vi "CRYUpdate Curve Name of All Steps.vi"(0 "Start Index":i32, 1 "sOption":string, 5 "End Index":i32) -> ()   [LabVIEW 2013]
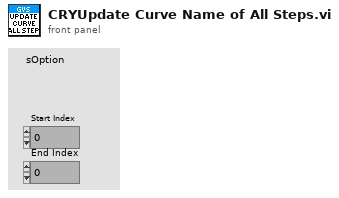
[diagram p1: front panel]
types:
  T1 = typedef "CRYStep.ctl" = cluster{"No.VI":i32, "Category":string, "StepName":string, "Seq setup flattened":string, "Comment":string, "Steps config.":bool[], "Jump config":i32[], "Start":dbl, "Increment":dbl, "Name":string, "Unit":string, "Y data":u16, "Y prefix":string, "Y dB ref":dbl, "Y unit":string, "Repeat State Array":cluster{"Start":dbl, "Increment":dbl, "Count":i32, "Num":i32}[]}
  T2 = enum16{"Curves", "Values", "Results", "WFM", "All"}
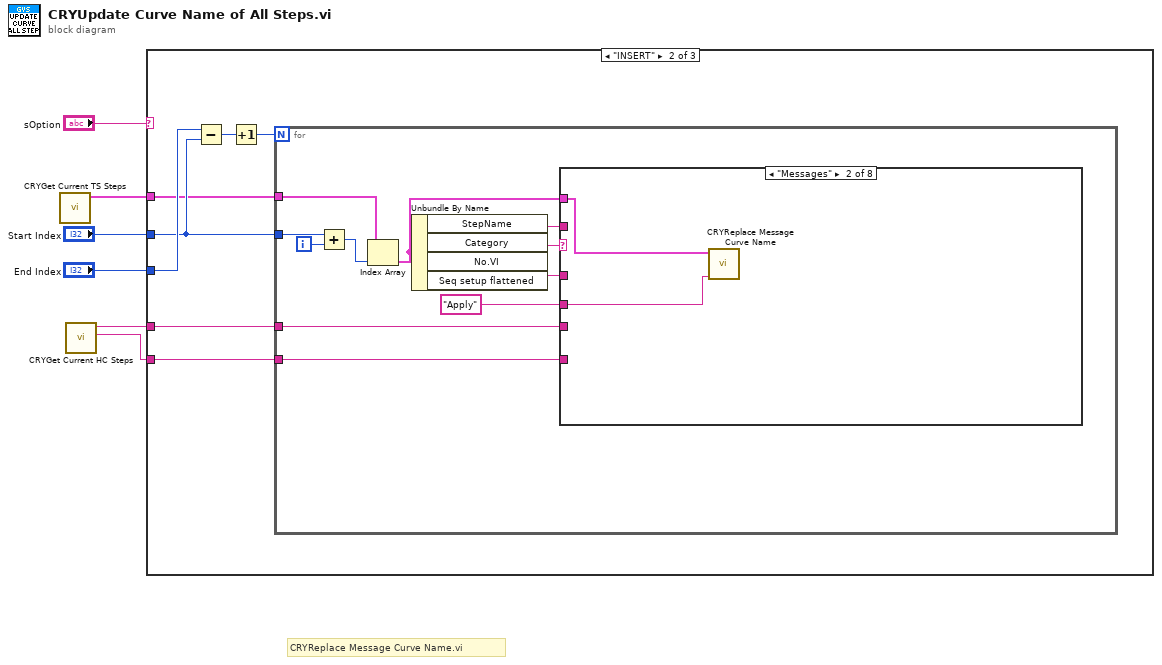
[diagram p0: block diagram]
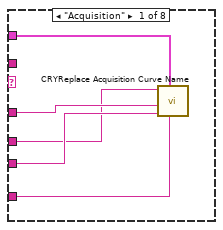
[diagram p3: hidden frame]
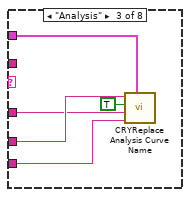
[diagram p4: hidden frame]
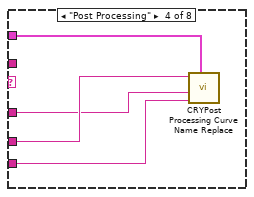
[diagram p5: hidden frame]
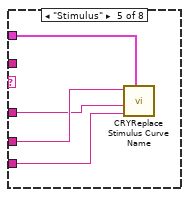
[diagram p6: hidden frame]
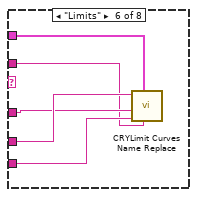
[diagram p7: hidden frame]
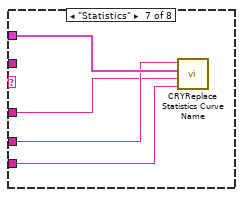
[diagram p8: hidden frame]
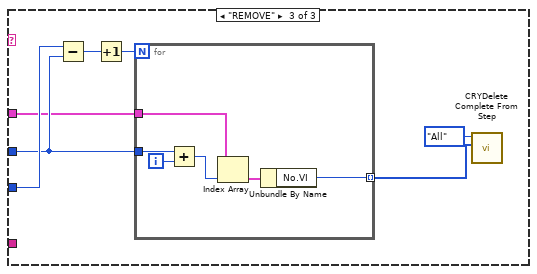
[diagram p10: hidden frame]
diagram:
  # "CRYReplace Message Curve Name.vi"
  n1 = call "CRYGet Current TS Steps.vi"() -> ("Steps"=w3:T1[])  [unwired: 7 in, 4 out]
  n2 = call "CRYGet Current HC Steps.vi"() -> ("Calibration setup flattened Out"=w1:string, "Hardware setup flattened Out"=w2:string)  [unwired: 10 in]
  n3 = case shown="\"INSERT\"" "sOption" {
    tunnel: "End Index" -> [_ w11 w58]
    tunnel: "Start Index" -> [_ w10 w57]
    tunnel: w3 -> [_ w9 w56]
    tunnel: w2 -> [_ w8 _]
    tunnel: w1 -> [_ w7 _]
    frame Default {
    }
    frame "INSERT" {
      n4 = Subtract(x=w11, y=w10) -> (x-y=w13:i32)
      n5 = Increment(x=w13) -> (x+1=w12:i32)
      n6 = for {
        N: w12 -> [_]
        tunnel: w10 -> [w24]
        tunnel: w9 -> [w19]
        tunnel: w8 -> [w17]
        tunnel: w7 -> [w14]
        i -> [w23]
        n7 = Add(x=w24, y=w23) -> (x+y=w22:i32)
        n8 = Index Array(array=w19, index=w22) -> (element=w18:T1)
        n9 = Unbundle By Name(w18) -> ("StepName"=w15:string, "Category"=w21:string, "Seq setup flattened"=w20:string)  [unwired: 1 out]
        n10 = case shown="\"Messages\"" w21 {
          tunnel: w20 -> [w29 _ w34 w38 w43 w47 w51 _]
          tunnel: w18 -> [w28 w31 w36 w40 w41 w49 w53 _]
          tunnel: w17 -> [w27 _ w33 w37 w42 w46 w50 _]
          tunnel: "Apply" ("Type In") -> [w26 w30 w35 w39 w44 w48 w52 _]
          tunnel: w15 -> [_ _ _ _ _ w45 _ _]
          tunnel: w14 -> [w25 _ _ _ _ _ _ _]
          frame "Acquisition" {
            n11 = call "CRYReplace Acquisition Curve Name.vi"("Calibration in"=w25, "Setup in"=w28, "Hardware Setup In"=w27, "Step Setup In"=w29, "Type In"=w26) -> ()  [unwired: 4 in, 3 out]
          }
          frame "Messages" {
            n12 = call "CRYReplace Message Curve Name.vi"("Type In"=w30, "Setup in"=w31) -> ()  [unwired: 10 in]
          }
          frame "Analysis" {
            n13 = call "CRYReplace Analysis Curve Name.vi"("Setup in"=w36, "Hardware Setup In"=w33, "Step Setup In"=w34, "InsertSocket?"=TRUE, "Type In"=w35) -> ()  [unwired: 2 in, 5 out]
          }
          frame "Post Processing" {
            n14 = call "CRYPost Processing Curve Name Replace.vi"("Setup in"=w40, "Hardware in"=w37, "Step Setup in"=w38, "Type In"=w39) -> ()  [unwired: 7 in, 1 out]
          }
          frame "Stimulus" {
            n15 = call "CRYReplace Stimulus Curve Name.vi"("Setup in"=w41, "Hardware Setup In"=w42, "Step Setup In"=w43, "Type In"=w44) -> ()  [unwired: 7 in, 1 out]
          }
          frame "Limits" {
            n16 = call "CRYLimit Curves Name Replace.vi"("StepName"=w45, "Setup in"=w49, "Hardware Setup In"=w46, "Step Set up In"=w47, "Type In"=w48) -> ()  [unwired: 6 in, 1 out]
          }
          frame "Statistics" {
            n17 = call "CRYReplace Statistics Curve Name.vi"("Hardware Setup In"=w50, "Step Set up In"=w51, "Setup in"=w53, "Type In"=w52) -> ()  [unwired: 6 in, 2 out]
          }
          frame Default {
          }
        }
      }
    }
    frame "REMOVE" {
      n18 = Subtract(x=w58, y=w57) -> (x-y=w60:i32)
      n19 = Increment(x=w60) -> (x+1=w59:i32)
      n20 = for {
        N: w59 -> [_]
        tunnel: w57 -> [w63]
        tunnel: w56 -> [w64]
        tunnel: [w62] -> w54 mode=indexing
        i -> [w61]
        n21 = Add(x=w63, y=w61) -> (x+y=w66:i32)
        n22 = Index Array(array=w64, index=w66) -> (element=w65:T1)
        n23 = Unbundle By Name(w65) -> ("No.VI"=w62:i32)
      }
      n24 = call "CRYDelete Complete From Step.vi"("Step No."=w54, "Type In"=T2."All") -> ()  [unwired: 10 out]
    }
  }
